vi "Waveform to Cluster.vi"(8 "Error in":errorcluster, 9 "Waveform in":waveform(dbl)[](array[waveform]), 10 "Label in":string) -> (0 "Error out":errorcluster, 1 "Cluster array out":cluster{"Y":dbl[]}[](array[cluster]), 2 "Output Label":string[](array[string]))   [LabVIEW 2019, in "Transport.lvclass"]
uses:
  Transport.lvclass
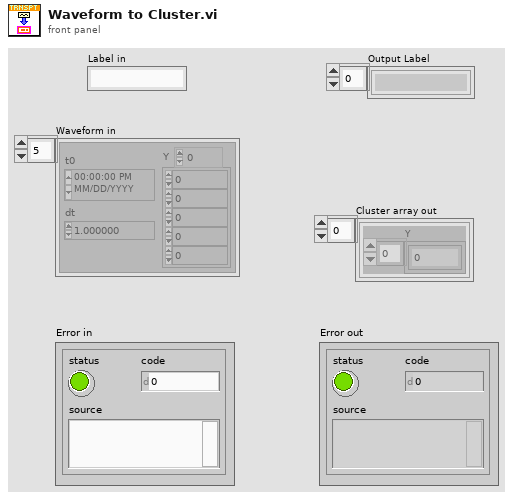
[diagram p1: front panel]
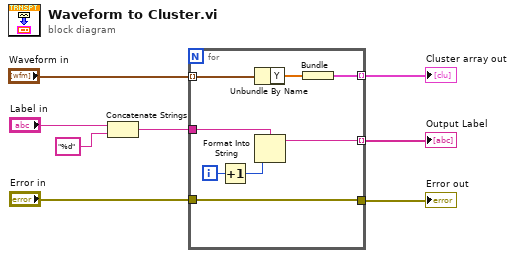
[diagram p0: block diagram]
diagram:
  n1 = Concatenate Strings("Label in", "%d" ("wavenames")) -> (w6:string)
  n2 = for {
    tunnel: [w15] -> w4 mode=indexing
    tunnel: [w13] -> w5 mode=indexing
    tunnel: w6 -> [w11]
    tunnel: "Waveform in" -> [w10] mode=indexing
    tunnel: "Error in" -> [w9]
    tunnel: [w9] -> w2
    i -> [w16]
    n3 = Increment(x=w16) -> (x+1=w14:i32)
    n4 = Unbundle By Name(w10) -> ("Y"=w12:dbl[])
    n5 = Format Into String(format string=w11, w14) -> (resulting string=w15:string)  [unwired: 2 in, 1 out]
    n6 = Bundle("Y"=w12) -> (w13:cluster{"Y":dbl[]})  [unwired: 1 in]
  }
  "Cluster array out" <- w5
  "Output Label" <- w4
  "Error out" <- w2
